vi "SaveToDropBox-XYGraph.vi"(0 "XYGrapf Reference":refnum<vi>) -> ()   [LabVIEW 2009]
uses:
  <vilib>/Utility/sysdir.llb/System Directory Type.ctl
  <vilib>/Utility/file.llb/Write To Spreadsheet File (DBL).vi
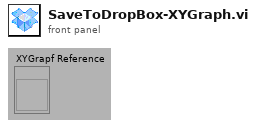
[diagram p1: front panel]
types:
  T1 = typedef "System Directory Type.ctl" = i32
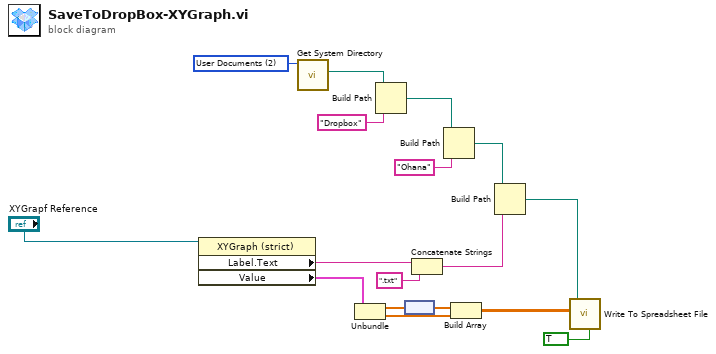
[diagram p0: block diagram]
diagram:
  w14 = T1 2 items=["User Home", "User Desktop", "User Documents", "User Application Data", "User Preferences", "User Temporary", "Public Documents", "Public Application Data", "Public Preferences", "System Core Libraries", "System Installed Libraries", "Application Files", "Boot Volume Root"] ("system directory type")
  n1 = property class="XYGraph (strict)"(reference="XYGrapf Reference") -> ("Label.Text"=w8:string, "Value"=w11:cluster{dbl[unit][], "Power Spectrum":dbl[]})  [unwired: 1 in, 2 out]
  n2 = call <vilib>:"Get System Directory.vi"("system directory type"=w14) -> ("system directory"=w16:path)  [unwired: 10 in]
  n3 = Unbundle(w11) -> (w4:dbl[unit][], "Power Spectrum"=w3:dbl[])
  n4 = Build Path(base path=w16, name or relative path="Dropbox") -> (appended path=w17:path)
  n5 = node(w4) -> (w2:dbl[])
  n6 = Concatenate Strings(w8, ".txt" ("string")) -> (w9:string)
  n7 = Build Path(base path=w17, name or relative path="Ohana") -> (appended path=w12:path)
  n8 = Build Array(w2, w3) -> (w1:dbl[][])
  n9 = Build Path(base path=w12, name or relative path=w9) -> (appended path=w7:path)
  n10 = call-poly <vilib>:"Write To Spreadsheet File.vi"("transpose? (no:F)"=TRUE, "2D data"=w1, "file path (dialog if empty)"=w7) -> ()  [unwired: 5 in, 1 out]
